vi "PathPlanner_GridPos_ToOccupancyGrid.vi"(11 "PathPlanner_Grid":T1 {"Field Size M"."Y" format="%14.3f"; "Field Size M"."X" format="%14.3f"}) -> (0 "error out":errorcluster, 3 "map reference out":refnum<data-value>)   [LabVIEW 2019, in "PathPlanner24.lvlib"]
doc: "Load a path from a JSON string.\n\nInputs: \n - JSON String - string- The string containing the path definition.\n\nOutputs:\n - Path - cluster - PathPlannerPath created from the given JSON string\n - Error out - cluster - Error cluster"
uses:
  PathPlanner24.lvlib
  <vilib>/robotics/Navigation/shared/WorldMap/OccupancyGridWorldMap/NI_Robotics_OccupancyGridWorldMap.lvclass
  <vilib>/Rock Robotics/WPI/ThirdParty/JAS_Junk/TrajLib/TypeDef/TRANSLATION2D.ctl
  <vilib>/Rock Robotics/WPI/ThirdParty/JAS_Junk/TrajLib/Trajectory_Library.lvlib
  TypeDef/PathPlannerGrid.ctl
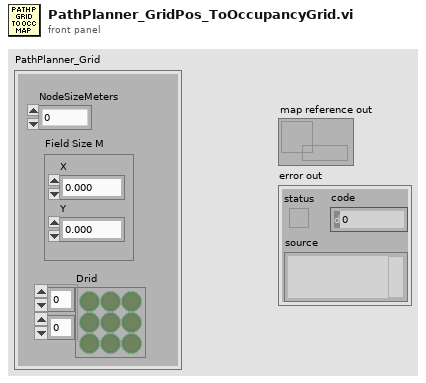
[diagram p1: front panel]
types:
  T1 = typedef "PathPlanner24.lvlib/PathPlannerGrid.ctl" = cluster{"NodeSizeMeters":dbl, "Field Size M":T2, "Drid":bool[][]}
  T2 = typedef "Trajectory_Library.lvlib/TRANSLATION2D.ctl" = cluster{"X":dbl, "Y":dbl}
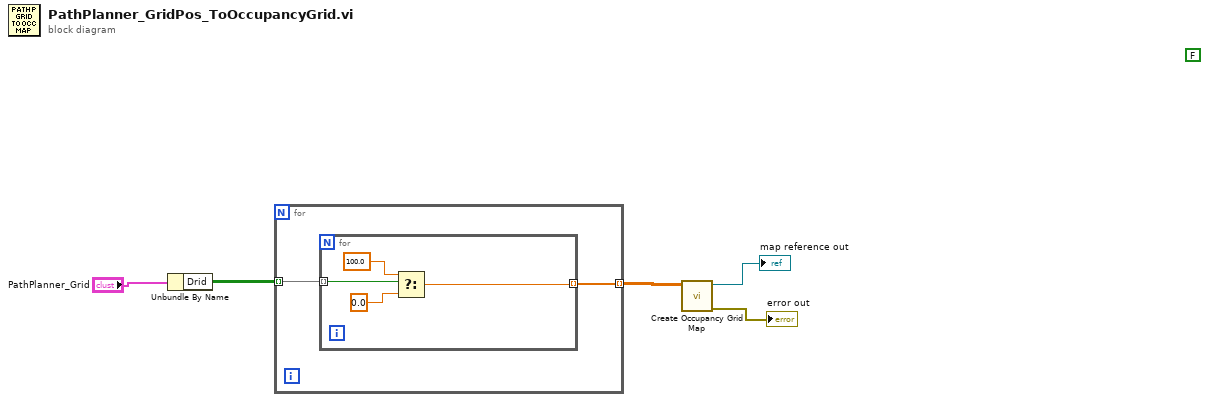
[diagram p0: block diagram]
diagram:
  (unwired) FALSE ("Error")
  n1 = Unbundle By Name("PathPlanner_Grid") -> ("Drid"=w4:bool[][])
  n2 = for {
    tunnel: w4 -> [w7] mode=indexing
    tunnel: [w6] -> w3 mode=indexing
    n3 = for {
      tunnel: w7 -> [w11] mode=indexing
      tunnel: [w8] -> w6 mode=indexing
      n4 = Select(t=100.0, s=w11, f=0.0) -> (s? t:f=w8:dbl)
    }
  }
  n5 = call <vilib>:"Create Occupancy Grid Map.vi"("occupancy grid"=w3) -> ("error out"=→"error out":errorcluster, "map reference out"=→"map reference out":refnum<data-value>)  [unwired: 9 in]
